vi "ExcelSaveArray.vi"(8 "error in":errorcluster, 11 "Mean":refnum<vi>) -> (0 "error out":errorcluster)   [LabVIEW 2017]
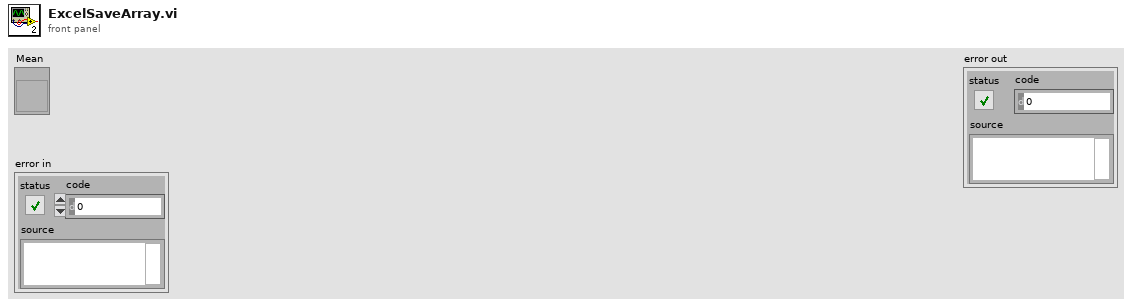
[diagram p1: front panel]
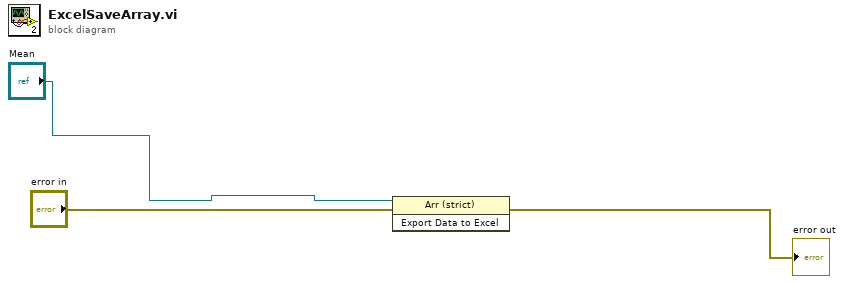
[diagram p0: block diagram]
diagram:
  n1 = invoke on="Invoke Node" class="Arr (strict)" method="Export Data to Excel"(reference="Mean", error in="error in") -> (error out=→"error out":errorcluster)  [unwired: 1 in, 2 out]
